vi "SetAccTimes.vi"(8 "错误输入（无错误）":errorcluster, 11 "指定的通道号":u32) -> (0 "错误输出":errorcluster)   [LabVIEW 2014]
uses:
  X86Dll/ZXUTConfigMgr.dll
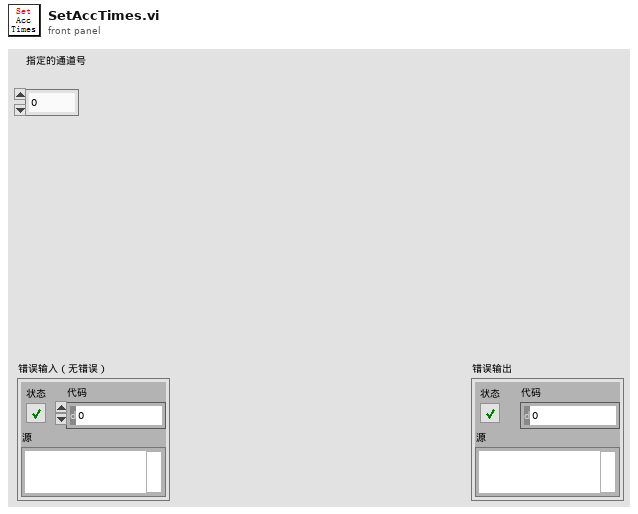
[diagram p1: front panel]
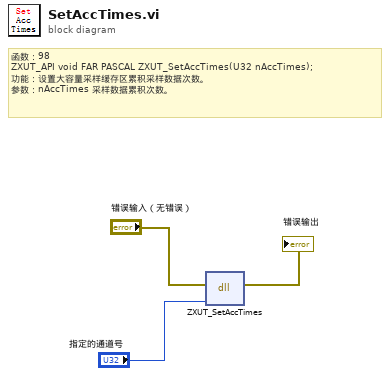
[diagram p0: block diagram]
diagram:
  # "函数：98\nZXUT_API void\tFAR PASCAL ZXUT_SetAccTimes(U32 nAccTimes);\n功能：设置大容量采样缓存区累积采样数据次数。\n参数：nAccTimes 采样数据累积次数。"
  n1 = dll-call lib="D:/Software/Utrasonic on-line monitoring/X86Dll/ZXUTConfigMgr.dll" fn="ZXUT_SetAccTimes"(error in="错误输入（无错误）", "nAccTimes"="指定的通道号") -> (error out=→"错误输出":errorcluster)  [unwired: 4 in, 1 out]
